vi "BoldDecorator_Create.vi"(8 "Error In":errorcluster, 10 "Text":refnum<class "AbstractText.lvclass">, 11 "reference in":refnum<class "BoldDecorator.lvclass">) -> (0 "Error Out":errorcluster, 3 "reference out":refnum<class "BoldDecorator.lvclass">)   [LabVIEW 2024, in "BoldDecorator.lvclass"]
uses:
  BoldDecorator.lvclass
  BoldDecorator.lvclass/BoldDecorator.ctl
  TextDecorator/TextDecorator.lvclass
  AbstractText/AbstractText.lvclass
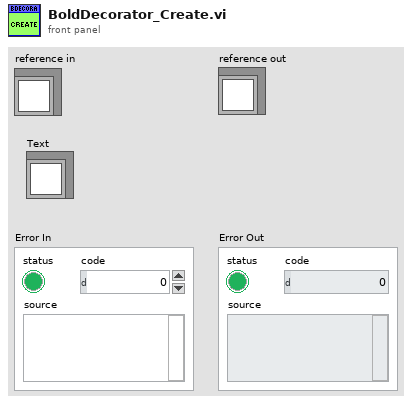
[diagram p1: front panel]
types:
  T1 = typedef "BoldDecorator.lvclass/ObjectAttributes.ctl" = cluster{"None":bool}
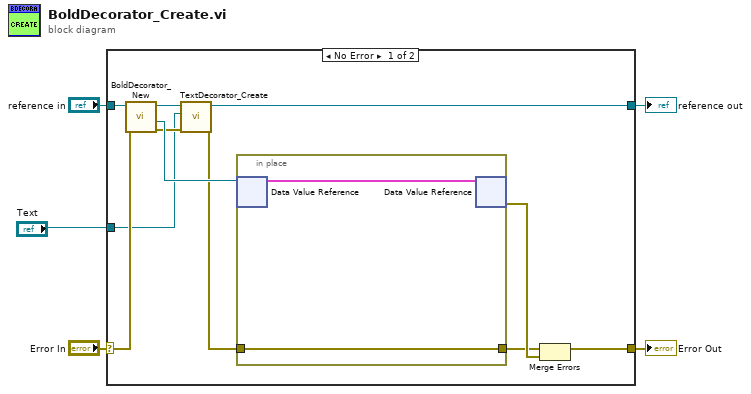
[diagram p0: block diagram]
diagram:
  n1 = case shown="No Error" "Error In" {
    selector: "Error In" -> [w12 w20]
    tunnel: [w10 w20] -> w4
    tunnel: "reference in" -> [w14 w19]
    tunnel: [w9 w19] -> w2
    tunnel: "Text" -> [w6 _]
    frame No Error {
      n2 = call "BoldDecorator_New.vi"("Error In"=w12, "reference in"=w14) -> ("Error Out"=w13:errorcluster, "DVRRefOut"=w16:refnum<data-value>, "reference out"=w15:refnum<class "BoldDecorator.lvclass">)  [unwired: 6 in, 1 out]
      n3 = call "TextDecorator_Create.vi"("Error In"=w13, "AbstractText"=w6, "reference in"=w15) -> ("Error Out"=w8:errorcluster, "reference out"=w9:refnum<class "BoldDecorator.lvclass">)  [unwired: 7 in]
      n4 = in-place {
        in-place-border: w8 -> [w17]
        in-place-border: [w17] -> w7
        n5 = in-place-dvr #1(w16) -> (w18:T1)  [unwired: 1 out]
        n6 = in-place-dvr #1(w18) -> (w11:errorcluster)  [unwired: 1 out]
      }
      n7 = Merge Errors(w7, w11) -> (w10:errorcluster)
    }
    frame Error {
    }
  }
  "Error Out" <- w4
  "reference out" <- w2
